vi "判断局域网内-是否存在指定IP地址的计算机.vi"(11 "IP地址":string="192.168.0.70 ") -> (3 "IP可用？":bool)   [LabVIEW 2013]
panel:
  out "传输失败？":bool
  out "standard output 2":string caption="标准输出"
  out "无法访问？":bool
  out "超时？":bool
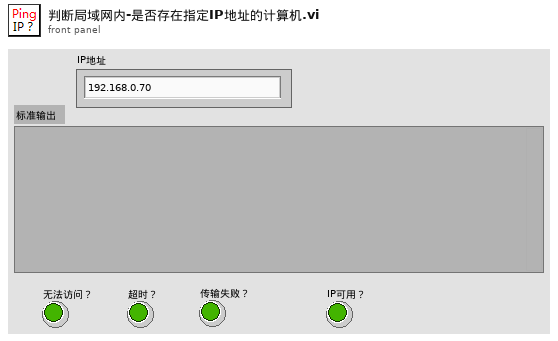
[diagram p1: front panel]
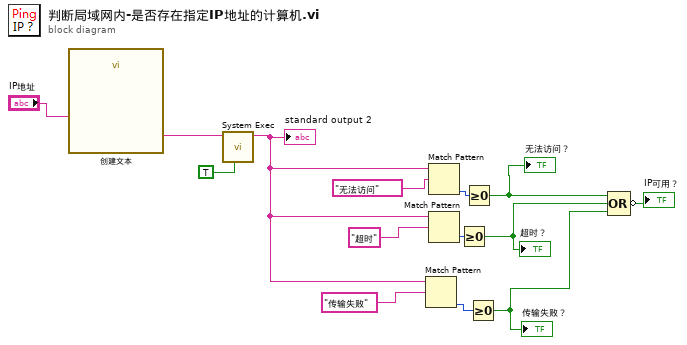
[diagram p0: block diagram]
diagram:
  n1 = call "创建文本"("IP地址"="IP地址") -> ("Result"=w10:string)  [unwired: 13 in, 1 out]
  n2 = call <vilib>:"System Exec.vi"("run minimized? (F)"=TRUE, "command line"=w10) -> ("standard output"=w7:string)  [unwired: 6 in, 3 out]
  "standard output 2" <- w7
  n3 = Match Pattern(string=w7, regular expression="传输失败" ("正则表达式")) -> (offset past match=w4:i32)  [unwired: 1 in, 3 out]
  n4 = Match Pattern(string=w7, regular expression="无法访问" ("正则表达式")) -> (offset past match=w6:i32)  [unwired: 1 in, 3 out]
  n5 = Match Pattern(string=w7, regular expression="超时" ("正则表达式")) -> (offset past match=w5:i32)  [unwired: 1 in, 3 out]
  n6 = Greater Or Equal To 0?(x=w5) -> (x >= 0?=w2:bool)
  "超时？" <- w2
  n7 = Greater Or Equal To 0?(x=w6) -> (x >= 0?=w1:bool)
  "无法访问？" <- w1
  n8 = Greater Or Equal To 0?(x=w4) -> (x >= 0?=w3:bool)
  "传输失败？" <- w3
  n9 = Compound Arithmetic op=OR(w1, w2, w3) -> (invert →"IP可用？":bool)
